vi "Init.vi"(8 "error in":errorcluster, 9 "Handlers":refnum<class "Handler.lvclass">[](array[class]), 10 "Name":string, 11 "Logger in":refnum<class "Logger.lvclass">) -> (0 "error out":errorcluster, 3 "Logger out":refnum<class "Logger.lvclass">)   [LabVIEW 2020, in "hse-logger.lvlib" / "Logger.lvclass"]
doc: "Initilizes a new Logger object and the specified name and handlers.\n\n____\nHAMPEL SOFTWARE ENGINEERING v2.0.6 (2021-04-15 11:38)"
uses:
  Logger.lvclass
  Handler/Handler.lvclass
  Logger.lvclass/Logger.ctl
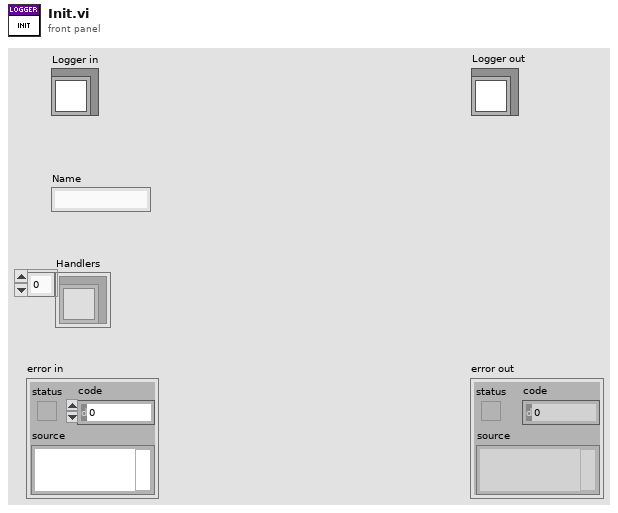
[diagram p1: front panel]
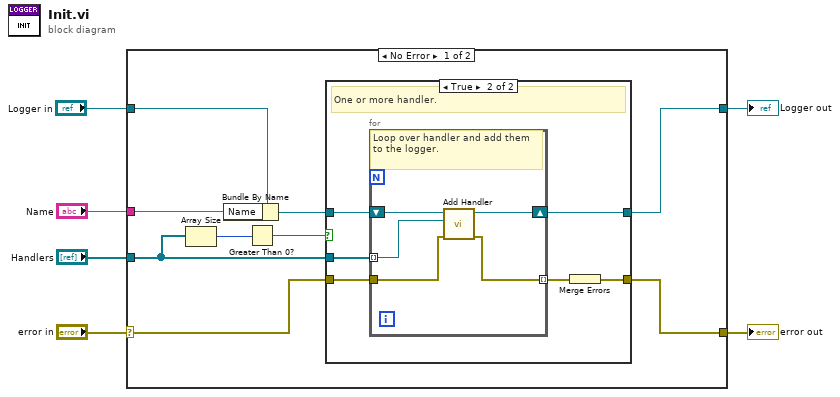
[diagram p0: block diagram]
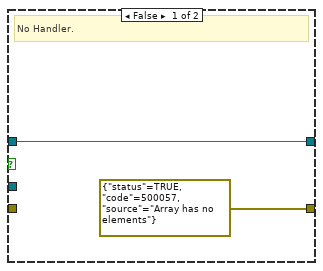
[diagram p2: hidden frame]
diagram:
  n1 = case shown="No Error" "error in" {
    selector: "error in" -> [w10 w30]
    tunnel: [w8 w30] -> w5
    tunnel: [w9 w29] -> w4
    tunnel: "Name" -> [w15 _]
    tunnel: "Handlers" -> [w11 _]
    tunnel: "Logger in" -> [w7 w29]
    frame No Error {
      n2 = Array Size(array=w11) -> (size(s)=w14:i32)
      n3 = Bundle By Name(cluster=w7, "Name"=w15) -> (w12:refnum<class "Logger.lvclass">)
      n4 = Greater Than 0?(x=w14) -> (x > 0?=w13:bool)
      n5 = case shown="True" w13 {
        tunnel: w12 -> [w17 w23]
        tunnel: w11 -> [_ w22]
        tunnel: w10 -> [_ w21]
        tunnel: [w17 w20] -> w9
        tunnel: [errorcluster {"status"=TRUE, "code"=500057, "source"="Array has no elements"} ("error IO") w18] -> w8
        frame False {
          # "No Handler."
        }
        frame True {
          # "One or more handler."
          n6 = for {
            tunnel: w22 -> [w27] mode=indexing
            shift-right: [w24] -> w20
            shift-left: w23 -> [w28]
            tunnel: w21 -> [w26]
            tunnel: [w25] -> w19 mode=indexing
            # "Loop over handler and add them to the logger."
            n7 = call "Add Handler.vi"("error in"=w26, "Handler"=w27, "Logger in"=w28) -> ("error out"=w25:errorcluster, "Logger out"=w24:refnum<class "Logger.lvclass">)  [unwired: 7 in]
          }
          n8 = Merge Errors(w19) -> (w18:errorcluster)
        }
      }
    }
    frame Error {
    }
  }
  "error out" <- w5
  "Logger out" <- w4
